vi "Register For Event.vi"(8 "Error In":errorcluster, 9 "Event Name":string, 10 "Registrant Enq":refnum<class "Message Enqueuer.lvclass">, 11 "Event Source In":refnum<class "Event Source.lvclass">) -> (0 "Error Out":errorcluster, 3 "Event Source Out":refnum<class "Event Source.lvclass">)   [LabVIEW 2020, in "Event Source.lvlib" / "Event Source.lvclass"]
doc: "This method registers a specific Actors Enqueuer and a Zero Coupling based message (inheriting from Event Generated Msg.lvclass) to used when the specified Event is Fired anywhere inside the Event Source Actor."
uses:
  Event Source.lvclass
  <vilib>/ActorFramework/Message Enqueuer/Message Enqueuer.lvclass
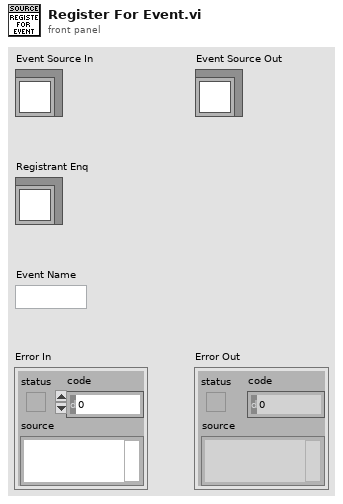
[diagram p1: front panel]
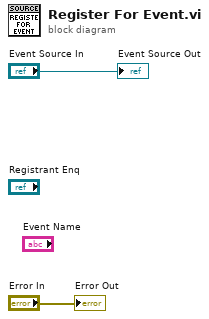
[diagram p0: block diagram]
diagram:
  "Error Out" <- "Error In"
  "Event Source Out" <- "Event Source In"
